vi "Cross Product Sub VI.vi"(9 "Speed and Rotation":T1, 10 "Module Location":dbl[](array[numeric])) -> (0 "Output Velocity (ft/s)":dbl, 1 "Output Angle (rad)":dbl, 2 "x velocity (ft/s)":dbl, 3 "y velocity (ft/s)":dbl)   [LabVIEW 2020]
uses:
  <vilib>/Analysis/NI_AALPro.lvlib
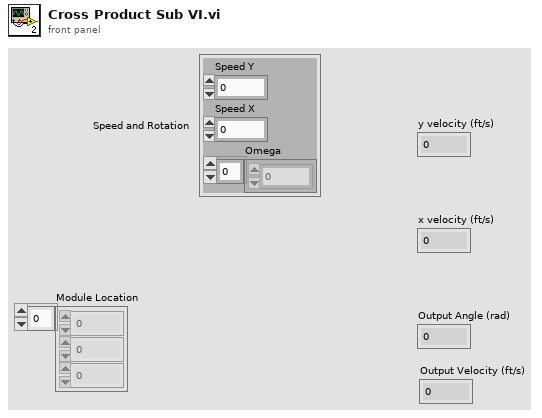
[diagram p1: front panel]
types:
  T1 = cluster{"Speed Y":dbl, "Speed X":dbl, "Omega":dbl[]}
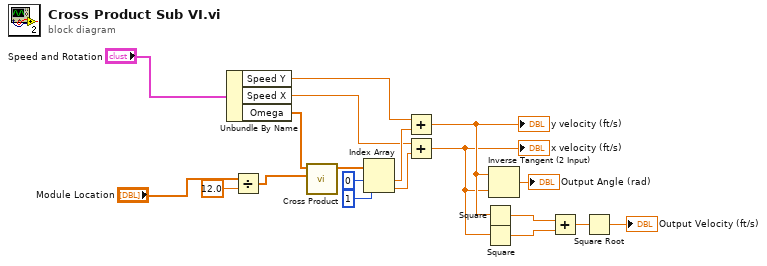
[diagram p0: block diagram]
diagram:
  n1 = Unbundle By Name("Speed and Rotation") -> ("Speed Y"=w1:dbl, "Speed X"=w2:dbl, "Omega"=w3:dbl[])
  n2 = Divide(x="Module Location", y=12.0) -> (x/y=w7:dbl[])
  n3 = call <vilib>:"Cross Product.vi"("B Vector"=w7, "A Vector"=w3) -> ("Cross Product"=w5:dbl[])  [unwired: 8 in, 1 out]
  n4 = Index Array(array=w5, index #1=0 ("index"), index #2=1 ("index")) -> (element #1=w9:dbl, element #2=w11:dbl)
  n5 = Add(x=w1, y=w9) -> (x+y=w19:dbl)
  "y velocity (ft/s)" <- w19
  n6 = Add(x=w2, y=w11) -> (x+y=w18:dbl)
  "x velocity (ft/s)" <- w18
  n7 = Square(x=w19) -> (x^2=w15:dbl)
  n8 = Square(x=w18) -> (x^2=w14:dbl)
  n9 = Inverse Tangent (2 Input)(1:w18, 2:w19) -> (0:→"Output Angle (rad)":dbl)
  n10 = Add(x=w15, y=w14) -> (x+y=w16:dbl)
  n11 = Square Root(x=w16) -> (sqrt(x)=→"Output Velocity (ft/s)":dbl)
